vi "TSM DAQmx Relay Configuration Control.vi"(0 "DAQmx Relay Configuration In":T1, 2 "Settling Time (s)":dbl, 11 "error in (no error)":errorcluster) -> (15 "error out":errorcluster)   [LabVIEW 2019]
doc: "Performs the actions specified by the relay configuration."
uses:
  Pin Map/TSM DAQmx Relay Configuration.ctl
  <vilib>/NI_TestStand_SemiconductorModule/NI_TestStand_Semiconductor_Module.lvlibp/PinMap/General/SemiconductorModuleContext.ctl
  Pin Map/TSM DAQmx Relay to Action Map.ctl
  Pin Map/TSM DAQmx Relay Actions.ctl
  <vilib>/NI_TestStand_SemiconductorModule/NI_TestStand_Semiconductor_Module.lvlibp
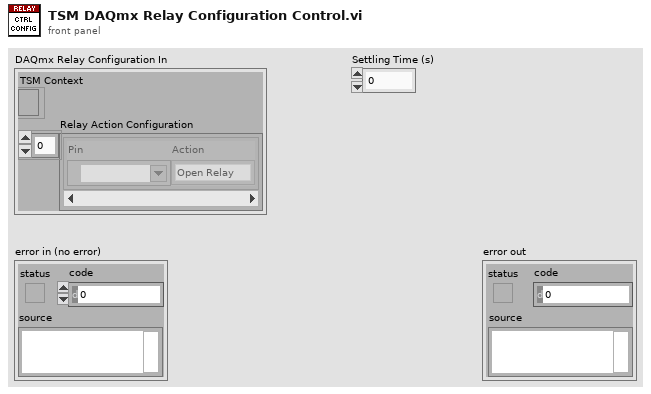
[diagram p1: front panel]
types:
  T1 = typedef "TSM DAQmx Relay Configuration.ctl" = cluster{"TSM Context":T2, "Relay Action Configuration":T3[]}
  T2 = typedef "NI_TestStand_Semiconductor_Module.lvlibp/SemiconductorModuleContext.ctl" = refnum<k7>
  T3 = typedef "TSM DAQmx Relay to Action Map.ctl" = cluster{"Pin":tag, "Relay Action":T4}
  T4 = typedef "TSM DAQmx Relay Actions.ctl" = enum16{"Open Relay", "Close Relay"}
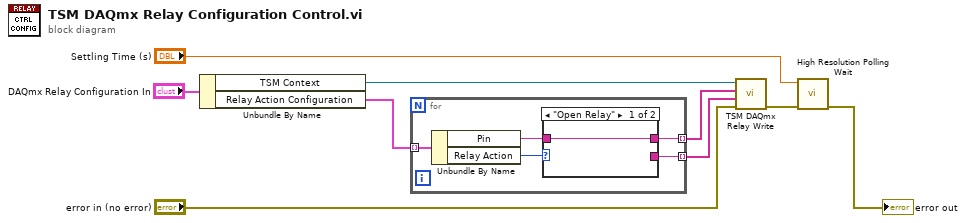
[diagram p0: block diagram]
diagram:
  n1 = Unbundle By Name("DAQmx Relay Configuration In") -> ("TSM Context"=w2:T2, "Relay Action Configuration"=w6:T3[])
  n2 = for {
    tunnel: w6 -> [w14] mode=indexing
    tunnel: [w11] -> w4 mode=indexing
    tunnel: [w10] -> w3 mode=indexing
    n3 = Unbundle By Name(w14) -> ("Pin"=w12:tag, "Relay Action"=w13:T4)
    n4 = case shown="\"Open Relay\"" w13 {
      tunnel: w12 -> [w15 w16]
      tunnel: [w15 _] -> w10
      tunnel: [_ w16] -> w11
      frame "Open Relay" {
      }
      frame "Close Relay" {
      }
    }
  }
  n5 = call "TSM DAQmx Relay Write.vi"("error in"="error in (no error)", "Pins to Output LOW"=w4, "Pins to Output HIGH"=w3, "TSM context in"=w2) -> ("error out"=w5:errorcluster)  [unwired: 6 in, 1 out]
  n6 = call <vilib>:"High Resolution Polling Wait.vi"("error in (no error)"=w5, "seconds to wait"="Settling Time (s)") -> ("error out"=→"error out":errorcluster)  [unwired: 9 in]
